vi "Select ILC Data.vi"(8 "error in (no error)":errorcluster, 9 "End Time":dbl, 10 "Start Time":dbl, 11 "Model in":refnum<class "Model.lvclass">) -> (0 "error out":errorcluster, 1 "StartIndex":i32, 2 "Data":T1[](array[typedef]) {"Timestamp" format="%.4f"; "Force" format="%.4f"}, 3 "Model out":refnum<class "Model.lvclass">)   [LabVIEW 2016, in "Model.lvclass"]
uses:
  Model.lvclass
  Typedefs/ActuatorData.ctl
  Typedefs/HPMT_Typedefs.lvlib
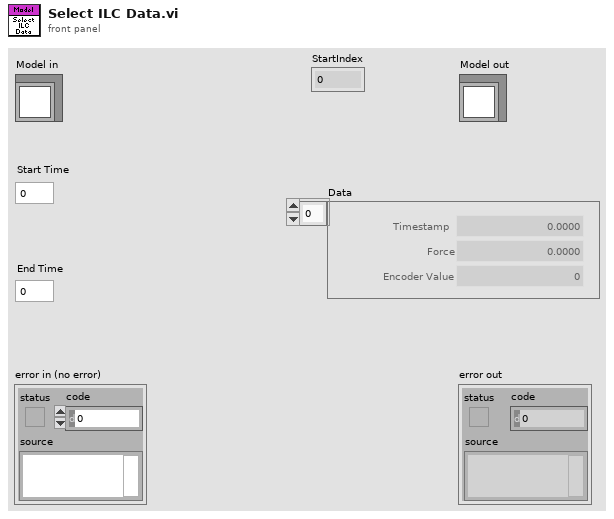
[diagram p1: front panel]
types:
  T1 = typedef "HPMT_Typedefs.lvlib/ActuatorData.ctl" = cluster{"Timestamp":dbl, "Force":dbl, "Encoder Value":i32}
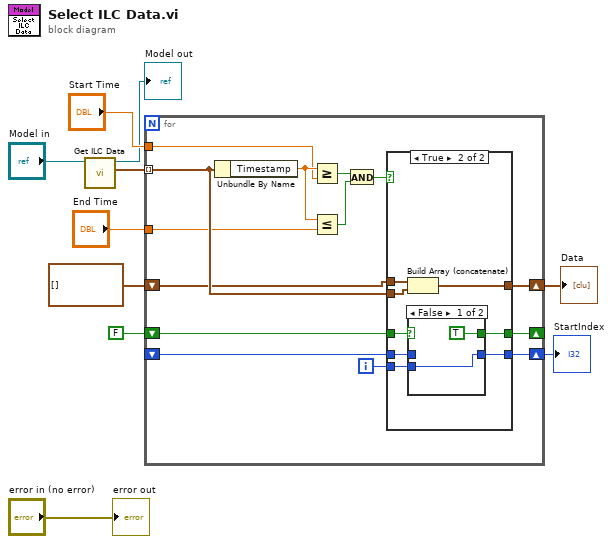
[diagram p0: block diagram]
diagram:
  n1 = call "Get ILC Data.vi"("Model in"="Model in") -> ("ILCData"=w9:T1[], "Model out"=→"Model out":refnum<class "Model.lvclass">)  [unwired: 9 in]
  n2 = for {
    tunnel: w9 -> [w20] mode=indexing
    shift-right: [w19] -> w5
    shift-left: T1[] [] -> [w18]
    tunnel: "Start Time" -> [w17]
    tunnel: "End Time" -> [w16]
    shift-right: [w14] -> _
    shift-left: FALSE -> [w15]
    shift-right: [w12] -> w1
    shift-left: _ -> [w11]
    i -> [w13]
    n3 = Unbundle By Name(w20) -> ("Timestamp"=w24:dbl)
    n4 = Greater Or Equal?(x=w24, y=w17) -> (x >= y?=w23:bool)
    n5 = Less Or Equal?(x=w24, y=w16) -> (x <= y?=w22:bool)
    n6 = And(x=w23, y=w22) -> (x .and. y?=w21:bool)
    n7 = case shown="True" w21 {
      tunnel: w20 -> [_ w35]
      tunnel: [w27 w34] -> w19
      tunnel: w18 -> [w27 w33]
      tunnel: w15 -> [w26 w32]
      tunnel: [w26 w28] -> w14
      tunnel: w13 -> [_ w31]
      tunnel: [w25 w30] -> w12
      tunnel: w11 -> [w25 w29]
      frame False {
      }
      frame True {
        n8 = Build Array (concatenate)(w33, w35) -> (w34:T1[])
        n9 = case shown="False" w32 {
          selector: w32 -> [_ w38]
          tunnel: w31 -> [w37 _]
          tunnel: [w37 w39] -> w30
          tunnel: w29 -> [_ w39]
          tunnel: [TRUE w38] -> w28
          frame False {
          }
          frame True {
          }
        }
      }
    }
  }
  "Data" <- w5
  "StartIndex" <- w1
  "error out" <- "error in (no error)"
